vi "Joystick 2 Grip System.vi"(11 "Secondary joystick buttons":bool[](array[boolean])) -> (2 "Close Grip":bool, 3 "Open Grip":bool)   [LabVIEW 2018]
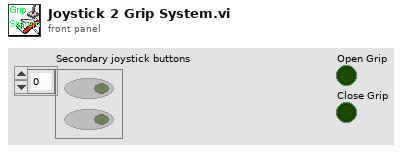
[diagram p1: front panel]
types:
  T1 = typedef "SecondaryJoystickButtons.ctl" = cluster{"Intake":bool, "Outtake":bool, "ShoulderMotor":bool, "ElbowMotor":bool, "Open Grip":bool, "Close Grip":bool, "Reset Arm Encoders":bool, "Eject Disc":bool}
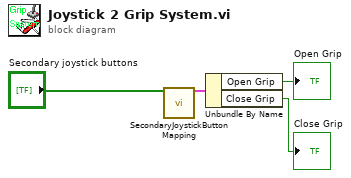
[diagram p0: block diagram]
diagram:
  n1 = call "SecondaryJoystickButtonMapping.vi"("Secondary joystick buttons"="Secondary joystick buttons") -> ("SecondaryJoystickButtons"=w4:T1)  [unwired: 13 in, 1 out]
  n2 = Unbundle By Name(w4) -> ("Open Grip"=→"Open Grip":bool, "Close Grip"=→"Close Grip":bool)
